vi "GetArrayLengthAndAddress.vi"(8 "error in":errorcluster, 10 "BytePerElement":i32, 11 "Payload":variant) -> (0 "error out":errorcluster, 3 "U8Data":u8[](array[numeric]))   [LabVIEW 2019, in "Memory Data Access.lvlib"]
uses:
  Memory Data Access.lvlib
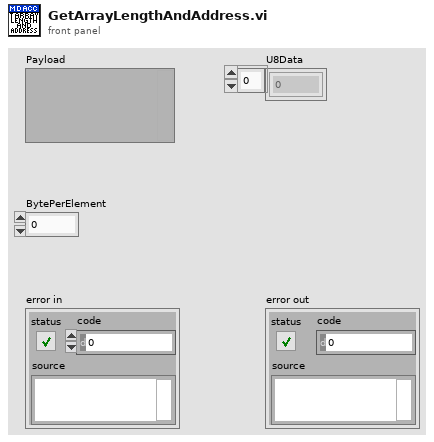
[diagram p1: front panel]
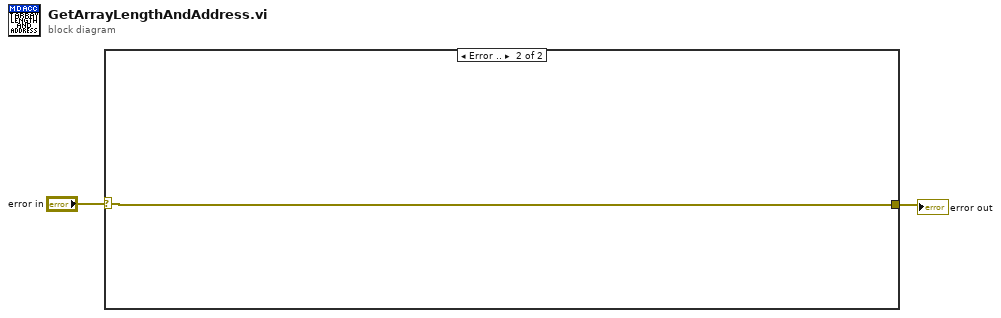
[diagram p0: block diagram]
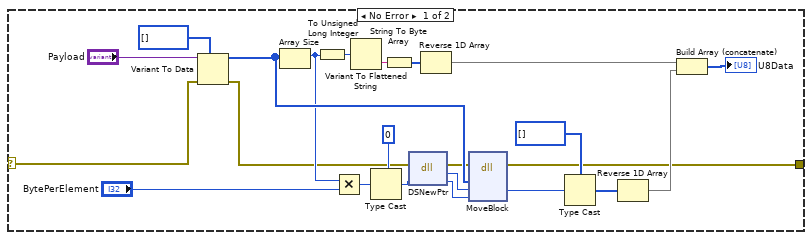
[diagram p2: hidden frame]
diagram:
  n1 = case shown="Error .." "error in" {
    selector: "error in" -> [w12 w26]
    tunnel: [w3 w26] -> w1
    frame No Error {
      n2 = Variant To Data(error in=w12, type=u32[] [], Variant="Payload") -> (data=w23:u32[], error out=w11:errorcluster)
      n3 = Array Size(array=w23) -> (size(s)=w19:i32)
      n4 = To Unsigned Long Integer(number=w19) -> (unsigned 32bit integer=w16:u32)
      n5 = Multiply(x=w19, y="BytePerElement") -> (x*y=w21:i32)
      n6 = Variant To Flattened String(Variant=w16) -> (data string=w15:string)  [unwired: 1 out]
      n7 = Type Cast(type=u32 0, x=w21) -> (*(type *) &x=w22:u32)
      n8 = String To Byte Array(string=w15) -> (unsigned byte array=w17:u8[])
      n9 = dll-call lib="LabVIEW" fn="DSNewPtr"(error in=w11, "size"=w22) -> (error out=w5:errorcluster, "return type"=w24:u64, "size"=w25:u32)  [unwired: 2 in, 1 out]
      n10 = Reverse 1D Array(array=w17) -> (reversed array=w18:u8[])
      n11 = dll-call lib="LabVIEW" fn="MoveBlock"(error in=w5, "PointerSRC"=w23, "PointerDEST"=w24, "size"=w25) -> (error out=w3:errorcluster, "PointerDEST"=w10:u64)  [unwired: 5 in, 1 out]
      n12 = Type Cast(type=u8[] [], x=w10) -> (*(type *) &x=w7:u8[])
      n13 = Reverse 1D Array(array=w7) -> (reversed array=w6:u8[])
      n14 = Build Array (concatenate)(w18, w6) -> (→"U8Data":u8[])
    }
    frame Error {
    }
  }
  "error out" <- w1
